vi "GOOP_XControl_Item_Init.vi"(11 "Object":u64) -> ()   [LabVIEW 2012]
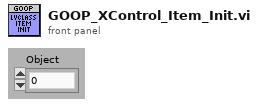
[diagram p1: front panel]
types:
  T1 = typedef "ItemRef.ctl" = u64
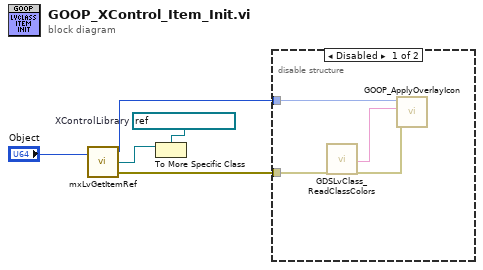
[diagram p0: block diagram]
diagram:
  w4 = refnum<vi> refnum  # XControlLibrary
  n1 = call <resource>:"mxLvGetItemRef.vi"("Item"="Object") -> ("Item"=w2:T1, "Item Refnum"=w3:refnum<vi>, "error out"=w1:errorcluster)  [unwired: 1 in]
  n2 = To More Specific Class(target class=w4, reference=w3) -> ()  [unwired: 1 in, 2 out]
  n3 = disable-structure shown="Disabled" {
    disable-tunnel: w2 -> [w8 _]
    disable-tunnel: w1 -> [w6 _]
    frame Disabled {
      n4 = call <resource>:"GDSLvClass_ReadClassColors.vi"("error in (no error)"=w6) -> ("ClassItemIconName(NoExtension)"=w9:string, "error out"=w7:errorcluster)  [unwired: 13 in, 4 out]
      n5 = call <resource>:"GOOP_ApplyOverlayIcon.vi"("error in (no error)"=w7, "IconName(NoPngExtension)"=w9, "Object"=w8) -> ()  [unwired: 8 in, 1 out]
    }
    frame Enabled {
    }
  }
